vi "Timeout.vi"(8 "Start Time In":dbl, 11 "Limit In":dbl) -> (0 "Start Time Out":dbl, 3 "Timeout":bool)   [LabVIEW 2014]
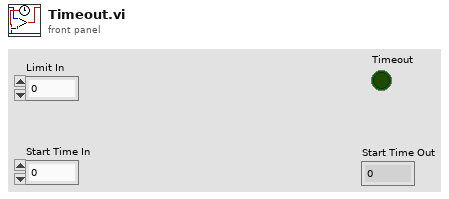
[diagram p1: front panel]
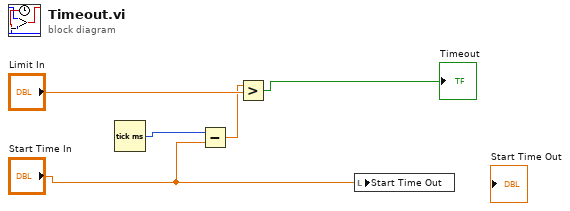
[diagram p0: block diagram]
diagram:
  n1 = Tick Count (ms)() -> (millisecond timer value=w5:u32)
  n2 = Subtract(x=w5, y="Start Time In") -> (x-y=w1:dbl)
  n3 = Greater?(x=w1, y="Limit In") -> (0:→"Timeout":bool)
  n4 = local write "Start Time Out"("Start Time In") -> ()
